vi "Parse.vi"(8 "Error In":errorcluster, 11 "object in":refnum<class "2024_19.lvclass">) -> (0 "Error Out":errorcluster, 3 "object out":refnum<class "2024_19.lvclass">)   [LabVIEW 2023, in "2024_19.lvclass"]
uses:
  2024_19.lvclass
  2024_19.lvclass/2024_19.ctl
  <vilib>/Utility/error.llb/Trim Whitespace One-Sided.vi
  <userlib>/_OpenG.lib/string/string.llb/openg_string.lvlib
panel:
  out "array":string[](array[string])
  out "Pattern":string[](array[string])
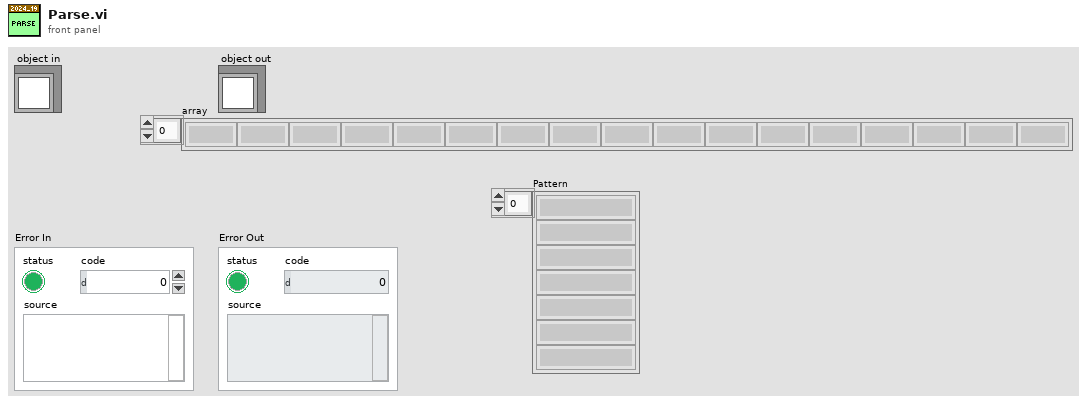
[diagram p1: front panel]
diagram:
  (unwired) "r, wr, b, g, bwu, rb, gb, br\n\nbrwrr\nbggr\ngbbr\nrrbgbr\nubwu\nbwurrg\nbrgr\nbbrgwb" ("PuzzleInput")
  n1 = call <vilib>:"Trim Whitespace.vi"("string"="bwwww, gwwug, ruw, wrbuwrbw, ugugb, rwwgw, wwb, ubgg, rubbwu, wgbuurbb, wrrbru, gwg, uuwwg, ugrrgr, uugrb, grwb, gwrb, buwrwuw, wrb, ruuggwr, rub, guwwr, gwrur, uug, ugguwru, uwr, rwuug, bwgw, ruu, wrbb, wub, wuwgugg, grgwrww, bgubw, wruuuu, bwg, wu, wbrbgr, bgwg, bgrubu, ggru, bgguww, rubgugrw, grwguu, wbg, ugub, urbwuurr, grb, ug, gbu, gbgwurbw, rrrburr, uggru, rubuwrrw, guwgrb, rbr, uruw, gggur, ugwg, bbwrr, ggbbbru, grbug, uuubww, rruug, ubbgwgr, brb, rbbuwbu, ggbrru, uuwugb, ubbgr, bubg, grbb, rgb, rwur, ubuuu, gwuwb, bubgrgr, wuuu, bwwg, urugg, wubuwubw, wgrb, gwggrgu, rwbu, bbbubgrg, rw, ggug, gwbgwbrb, bgugww, ggurrwg, rbbwuwu, wgw, bwb, bbw, urru, ugg, uwguu, wggw, wgr, urrr, urguwr, bbb, bgwbgub, guw, gu, gurwr, rgw, wbb, wggu, brbbg, wbw, rur, gub, rrbbr, uugruww, rbbrb, bwgrgr, rwrurww, grurg, brur, wbr, rgu, gguwr, bwurb, grguw, wuu, rwu, ubu, wbbwwub, urg, rww, bgg, wrwg, ugr, uru, urwggw, buwur, bbrgbwgr, bggbbgw, bbgu, rurrr, ugww, uurbur, brbw, wgwrbr, wbuuw, gwgu, rbw, gbwugwb, gbw, bwwgwr, wurrgwu, wwbg, rburuu, wrruwg, gg, bbbwugg, g, bg, wwguuu, gruwgu, ggrr, ur, bwwru, rwgub, rgwuu, wur, wuwrugw, uw, bubggbr, ubug, gwbbrw, rubgwg, rwbuub, rgrbugb, rbgb, wwgb, brbgw, uwwr, rbrg, uwrrur, uuwb, wug, bwwgrgb, rg, wuwww, bgrb, uurgw, rrburg, wubg, rwrwur, rwb, wrw, bwrw, wg, wwgrubwg, bugb, uuubguuw, gruu, wggruuu, urwu, wuugb, rrwww, bwrugbrb, wrgg, bru, ggww, wrbrrg, ugbu, rwwrrguu, wrg, buguu, ugbbww, urwur, grr, uuw, rrub, rb, bww, wgwr, ubb, bbbuub, ggbrw, rbwb, ubw, uuwg, wgrrbr, grw, gwu, wuwwgr, rwuw, gbbr, bguur, gwgrrw, bbu, ggg, grg, urbwwrr, bwgbuw, bw, gbrw, wbwrb, rurg, uurg, guugb, uww, brrbggbu, ruww, ru, rwguw, wgwbug, wwu, wgwwbur, bu, rguu, uwwwg, rug, wwg, brg, uwu, ubr, burg, ruug, rwr, uurugu, gr, uwubu, rr, rbwrbw, gw, uwwuu, ruuwb, rbg, wwrw, wruubg, bgwgrwbr, wuru, ggrgr, br, rwuu, grgbgg, urw, uub, rgrbb, wbuwb, wgwbg, ubwu, gwb, uu, rrrr, rru, gwr, uuubu, grgw, gbb, gwug, wbggwu, gggr, wr, wuw, wgg, buw, gbuwrwu, gb, uwb, bgubgb, rggbbbu, rgubgggr, rbgr, ruwr, wwr, grgbrb, ugrubr, ubgu, ugw, ugrr, ubg, ubgb, urb, wgb, wbwrbw, rugrr, ub, gbr, bugrg, ugu, rgrw, rrrrurr, bgbw, wgwg, guu, wrrubu, www, wrbu, bgrguwr, wwur, ubgbgug, wbwu, buu, gbgubrw, b, ggr, rrg, wwwb, wgrrrw, ubgrug, rrr, ugbb, wugubbur, bgwb, buwww, ugb, buub, wbrru, wuwguur, gwrggg, bgb, gru, bwwr, bgr, gbbw, wuruw, gbrgu, uwg, ubrg, ggu, bbwg, ugrbug, bbr, r, ugbwub, ggb, bbg, bggwb, bub, gbg, burbr, brw, wbuu, gugbb, uwubg, gbgwr, bgwwru, rgugb, uubgr, bb, gug, rggb, wugub, wrgu, wrwguug, gur, wru, bgbr, bug, bwu, ubbur, uurugb, ubgug, bgrr, bgbb, uwbrrug, bburur, rgr, brbbrw, rrrrwu, rgg, urwuwr, wwgr, bur, rugwg, bgu, urbg, wwrgbuw, rrgwrbb, uuu, grwgg, bwr, wrbrb, wrr, uwuuur, rrubu, ugwrg, rwuwg, wgu, rwru, rrww, urr, rwg, bgw, rbb, bgbubrg, bwbb, u, wggurggu, bubgw, ggw, gugg, ugrru, wbu, rggrrb, ubrgggwg, bwuu, rurb, wgrrg, brr, rubr\n\nwbugbugbgrgwubgrrgrubgbwubugrbrrubgwggggubrrrwrbr\nwbgrbrgbwrrurrrguwbubburbrwgwrbuwrbwgwuwubwurggbrggbr\nurbrbuwgbgwwwbgbwrugruburguwgwbgrugwrrbwbubgrwgww\nrrbgwgrwbrbuubbuugrurgbrbrwrbrggurwgwrbuwuwgubuwwrru\nuburbwruugurrbwbgbggrgrrurrugwuwggggubuwugbgurgugurbbbu\nwbubwwubrurggrrbbbuuwuwgggbguubwuubbwggrgubwbuggrbrrubg\nbbwbgggrwrrbwurubbrgugrguwrwwrrguurwwburgruwrrbrrbwgbggw\ngugrgwgbbwguuwbbrgwrruuuruwgbrurwubggbubbgrugubgbuwwgww\nbbrbbwgwwwbrgbrrgwgugwbwwrrbbwwgrwrrrrwwgrbguububgwrgww\nubuuuwrrwgwwgbguuurrgwrbbuggruurbwuwrubuugrwuuuwbwgubbuwgww\nuwuuwwwrrruggbbggrgwbbggwgurruwwgrugwrgww\nubbbrbbgubugugggugrbwuwbgbbruguburwugrubug\nrwwruggrwguwguwgguruubrggbgbbubwwrbbgbwbwwbbubbruwb\nbrubrbrurrbugwgrgrruuurrbgguwuwubbggbwgurbbuwugur\nwwrguwbwuggubgbrgbguburugbbwugrwwwggwwgbrgwrugrwuubgwwrggw\nuuugwubwgwrbuurbrwuuuubwgbubwbwrgbgrrbbggrwbwbg\nbrgbbrugbwbbwbuugubwrbuggruubrgwwuggugbubbgub\nurbrwguurgbbrgbwrugggwwgwubbguwrurbwburrwgu\nuwrbgggguruwubgrruwrguuuubwugwwrgbgubwrwguubuubwugwbw\nguugwbgwbrgurbrbwwrrubbbuurruuubburgrruwguwwwww\nwuugwbwbrgbgubgwuwwbggbubrugubrgggwgrrbrrrbuwgbb\nwgwgwurrrbwbwuuwgbwrggwruuuwbuuuuwrrbrrbbugwuubrwu\nwrbbgbbgugbbwwurruuruguuwuwbubbgruwurwruggruwbrbbwbwwbu\ngwbgwbbwwwuubrubguggguwbguuwrubwbrgwwugwbuuwurwrgurub\nugubrbubwbruubwugugrrbwbuggbgbrrgbrrgbbbgrguwwbrgww\nugbbburwwwbrrbrwbrwwbrwwubrrrwwubwgrrrbbgrwbbub\nuuuwgbgbuwguururugrbbbwuwurbuubuggbururrgbwuwwrwuuguuugwgww\nrwrbrgbuggwwbggwggrrwbgggwggurrbwbbubrgbuggbbrrugrbwwuwrrgww\nbrggrbgbruwrggwbbbuwubuwgwbrwgrwrwrwruuwggwrruwgrbru\nbuwugrgrbggwrbuggbubwwugugggbbrggwugbugburgrrbgbuwr\nurrwwwgwrbgwgbuwrggggrgbburwgwuuguwbwrrbbwwbgbwrwwwwwgrgww\nuwwbgwbbbggwbbbrgubrrrgbwwrwwbwbuwurubgww\nbbrrurwwggrbgwggrrggrrgugbubwuwbbwrbrgubgggbgu\nwbuugbubuwbrugrwgwbrrgggrubrbrwbgrgwgbrwubgrgww\nggugbrggrrbrgbbwguuruwurggbbggrbugbgwrbwbugbwwuurwgbbggwub\nurbwbubwurrgrruubwurbwwrwuwguurrrgbwgbwguwrgbgwwrwrugbbw\nbbrgwuubwrgubbrrgrwgugbrbuwuwuuurwgwgbgrbubbbruuubgwg\nwwbwbbbwurgubggugrbwrrbwuugugwbrrwuwbrwbrrrbrwbbbgrrrwgwgww\nuwwubwgubbwwugrugbwrugwbrwrrwbbgbugruwbwggruguubbrw\nuuruwbgwbwbrggrbgrugbgwwbbbgugurgrgggurbwrrwurguu\nbrbgrruwguugwbuwubwwbgwgbugbgrubrbbubbwubbuggbrgbrwugbrwwgww\nbrwrbwugubuguuuggrurbwruugguwugwgugwrbrbgwwrbwuurwwuur\nbbbguugubrugurrrgugggwbrrrgrggbugwwurrgrwuguwgbwrbgwgwg\nburrrgruugbbugrwgbrwrrgrugwrwrgbrrbgwwbbuubgw\ngurrgwuubbruwuwgbugbbbrwuwgbwurrurrugurruugrgbbrb\nbuwurgurguguuuurbrrwgwgbgbwubrgrrrgbrbuwggwrurbggurb\nwbgwgbgrgbwubwgubbbbrggrwwgwuuubbbrbwburgww\nbgrugwbgbwwwrugrgbbwwrrgurrbwurwurggwbwbbwbruu\nwbrwggwrwbggwwurwbububbuwbwwuwwurgggwugbbuwgurruwg\nububrrrruwrwburrggbgwwbururuwuurugrbrrrwrbgbb\ngbgrwggrguwurugrrrbbbubwrugrwubuwurwuguggwwrbr\nwgbguuwbbrrrgruwgugrgrwgrrugbrgrubugubggbrbwwrwwwwguwugu\nrwuurububuubburbwwbbuubbrgrrbubbwgbwrrguwrrbubrgggwgww\nrrrburbguwrrgrrbgrggggrbwgrbgrwbbbggugbubrw\nggrwgwubbuwrwruwwgwwbbwbgbwggubwgbrrubgww\nugwbbwgubbwurwbbrrbubugbgwwbubbbrgbwgrugrbrrbwgww\ngrwwwggbwuwrguugrbgrggbubwbbgguwuguurbwgubwuguuwrggwwr\nbrrwgbuurugrbuwguwuurguwbbwgbwbrwuubruwubwgbgbg\nubrgbwruwguurrburgururuburwwrrguurubuugrbbrbggrwbuuuwrrgww\nrbwgguggbrbgbgwgrgrggbgbuwbgububrruwrbrgww\nggrgwuruurgbwururwbbbrbbubgubugwubbbwrurgburg\nguuwbwgwurbrugggrwwwbrwrbbggwgugwubbubgggu\nwwggrbwgbgbrwwuwbwurgwbubbggbbgwrrggggrbwgugb\nburgburgggbgrwbrrrbgwgbwwbubgwwbugubgwgbwwrrwwwrrug\nugbbbrwbgruuwbwwggbwbguubrrrbgbbwbbbgburbgww\nuuburguubgubgggwbwggurgguwbbrgbubwuguururrbwrg\ngubwuwubrwgugrwwwuwbrgurrwwbrggrbwbggwubgrgruw\nguwgrbruruwrbwruuwggrwwwrburgrbggbwugbgww\nurwubuwuruubggwwggwuwwggrbrgburwrbruwrbwrrgww\nuuruugbuururbguururbgbugguuuuwwgguubwruguwwgww\nwgrbguguwgwbguwwbwrrwrwgbubrgurrgwwgwruuggwbwubb\nwburburwbgwrwgwwwrwggrwwurrbrrruugurgubrgg\ngbguguwwburwgburrgrbgugwgrwrwruwubugbbgugbwggrrrgww\nuwgwbruwuurgwgrgbuugbgurwruwrbbugggbbuuwrbg\nubgbwbrrrbwuruurggugwubruwwgurwgbbggwbbwrrwburbb\nrgwuuggrurgwwuuuwrruwggrgbwwbuwwbbwurrbggwrwwurrwgww\nrbgubuwrwuwrrbbuugwwurruugbuwguwugwrgrgbwburrwub\nrurbrrwugbwgwrrbwbwrrubgwrugbwwuggbubwugwrwbuuggbgrrb\ngrbwwgbrwrurwbwrbgrwrwuwuwburbrwbwugwgwrwgggrbuwb\nugurrgguwbbgbgbgggbrgwbrwwwrbubuurbbwwbgrgww\ngubuugurbrrburwgruuuwbbruwuubuggwwwbrwwwbwwrrggwb\nugurrbrgwurgrrwubbgbwwwbgurrruruwrbwgbrbrruuwuwgwwwbgrggbgww\nbwurwubwuruwggguwugrrrbwrubbgbuguguwggbwubrwurbwbrwbugwbu\nrwubrbbbuuuwuurrbgbugggwbbgbgwurbuuwbruurguggbuuwrrrubwuug\nwrgwrrwguggbrwrbuguruwwrbbbwbbwgbwubururubwrwubrw\nbuwguruwgrwrwwrbgbbrrbggbugwrrugrburubgbggrbbwubwbgguuwubgww\nwwubrbrgwrburbruurgurrgrbrwbrbuwugurbwuubwgwrgbuwu\nrbwrggwgbrbrrgbrwuwrrrrwurbggwwuwubuugwbugrguubrw\nuruggbgubbrrgbrbwwguurggbbugugrrggubuugwwu\nggbrwgbbggbwgwggbbguurgbgbbbubugbbgrugrgubbu\nggbggwbbrgurwrrrgugbgwbgwwwugguguuugrbuwbwbwbrbbgbrbgwur\nrbwrbugwrwwwrwwugbbrbrubrrgrugrwrwgbuubuwgwuwgrrrbgww\nwgwwrwgwruwgbbbbwgbbgbwgwrwruwwrwwuuurgrwgww\nwwgbbuwguuuwbrubbbwrrgbwwrguuggwuubuuwubbruw\ngbgbbuwbrwwbrurgwbugbwuwurbugbugwrwgwwbwwuwuwbuuuwr\ngbwubuuwurbuwbwuuguguwbwgbgrbgrgburubwbruuub\nrwwrgbrrbrbbbrgrwgrgbgwwgrwbbrrguwbwwrgrruugrrgww\nwrbgbrgrwuwwgwrbrgwbubwuwwguuuwurgbbrwgwrruwgg\nuwrbgrgruwubggrgrguugrgubbwrbwwbubwgugurrbgwrugbgw\nbugguuguwbrurrbrggbwwguubrggguuuwgggrbbgrgbrubbrrgrugwwrg\nbgwrwbuuwuuwrruwgrrwbuwuuruurgrbgurruwruwr\nurrrrbwrrgbuubrbbgggggubuwbbguuwurwgbrbgww\nrrbgwubrwbwbuuuguuguubruwrurggwgwgrrgbwbrwurbwbwgrwrgurwwg\nwrwurgwrgwgwwuurgrgggguwbgrwuwbwbwrgbbbbguugbbrbrruguwgww\nubwwbugbwwwrrgrbuwbbwuwubbggruuwrbugruwbrbbbubrw\nrrbrgggubrbwrrwrwbuubugrwbgwrurbugubwbrubwrbrrbwwbr\nubwbgbgubwgrbgubrbrgurrgrwbgrgrgwrugbwuuwgwuguwwugwgwururg\ngwwugugbgwbgggwggwwuubwwurwbbbrggbuuwgbrrggwbwwbbbgru\nbgwgbbuuwbrrgrbbuwwwwrwugggrgwrgbubrgbwgrgwgruwuuubgrw\ngruurgugwubuwbbbrbgrgwbgrgggrrbuwrbuwbruwwwurbbr\nrgrwuwbwbruwwrrwbgwwrubuwrrwrrbbrrugrubbrgbwwurbrwwgww\nbggwwrrurwugurgrwwwbrrggrrwgwgwgrbuuubuguw\nbbgbuugrgwruwgwubbrbuurbruwwwgwbrugrgurwbgwugwwbrb\nurbbggbrurrrrbrbbuuugwgggbggwugggbwwbrgbbrubw\nbgguuwrgrwurgbwwubwrggbbggrbrrurwbgwrgguubgurrggrgwbggbg\nrgbuwrurggubbugwbubrrgwbbbrubuugubbguwurwguuuugbu\nurwuwbbgrgbwggbrbbbbbrggbwwwgrurguwrgubrgwrbwbgwwwgww\nbubugwgbwwuwwurrrbububwuwbgbbggwubrbbuwugrwuburgrwgbugwr\nbrwbubwurgwbggguuwurrbugurrugwrbbbwggbgww\nruguwbrrrbgbwwuuwwbgrwwugrrbuubgrwburwuggubr\nrrbugrbrrgwruugrgbrbuggbruguwbwrubbruubrrrgbgrgwgbgbb\nbugggurrrrrgbuwbggbwgrgrrbwrgrgrgubuwwurbbwrggrwruwg\nrwrggruurbwguuguwbbrwwgrruguuwrrugbbggwgbbuububur\nbrbggbwwgwbbruubuguguwbruurugwrrgbgbwwgubguwrwuru\nwgwurwruruburruwwwgbgbbwuuwbwgurrgwurwbbwrrwwu\nggubruuuubggrgugubugrgguwwgguwwwuruuggubbuwrru\nbbbggwrbbgrwuwwbggwrbwbrwrguwgggbwbbrgbuwrrb\nwrbbgwgugrggbrwwwbguurwrgbrrwbguuugwrbwubbgwwubrr\nbbgbuwurgbgrrwbuurwbgburgwwbbubwggubrburbrbgwrrbwrbuwgug\nruuwrguruburruwwrugbwwrubgrgrruwruurwwwgrgrurr\nrbwwwwubwrwrurbrrwuwwbgruuurbwbrwgbrbubgwuubwurgww\nugrbgubuuwwwrbggrrwbbuubwgwbgwrubwgubwubuwubgwuubwruwu\nwwwwbbrgbwgrugrgwrgurwwuruubrubgwugwwggrrgg\nwbwbwbrwuugburwrgbrbrbwgbwbgwwuruurwbrbgwuuwbr\nuubuurwgbrubbbwbgrrrrwuuwgwggwgwwuggggbuurgguuwgw\nbbbrbgburggubrgruggggubbbubugbbrgrguurwbugb\nurrrwbgrburwuwuguwbrubwgbrgrwgrbrbuwggurgguwrgrugurbwgww\nwuggrrwguwwuruugrrbwwgugurburgugurwgrbwbuuwwrubgwgbwuwu\nbrrrgbrrrwbrwrbgggbbgwgugwruwrwgbbrwwbwrrbgbburgww\nwbuuwgbguurgbwuuruwbgbwuuuuwbuggbwwurbwubgwb\nuggrrrgwbrgruwrwgugbggwgrwrbubburugbwuuwrwbgugwwbwrguwrwrgww\ngbwrrbuguwwwubuuguruurbbwbwbbuugwurwwgbuurbbwugrubrbubbgww\nbgrrwruwrwbbwgwuwruwwgbbrwgburbrrrrwwwuwrbgrrbrwuubgww\nubgrgwrgurbgwgwwugbbbrrwgwruuurrwbubwwugurgwggg\ngrubgrbgwrbbbbbubuwwrwrurrbbrrbububwwwwuuub\nrbwrburbgbrbrgwwuwwbgubrrguurwugbugbuggubrwwururrburgurgb\nwrwgurbrwgwgwrwugrgugrwbgbguugbbuwrwrrbwggbbgrgwuu\nguggwgbgwurbbrrwrwwggrwwgrbubgurgwwwgrgbwwbrwwuwwwrruurr\ngrwubwrrubwwgwbrgbrwwwgbbbgwurrbbrrgurwwuwwubwbgubuubugrrgww\nurgggugwgwurwwbgbbrwbuggwrggbbbbbwuggbrbrruu\nrbuuwwwurugubgbgubggbwbwrrrbbbggbgwggggguwwrrrwwr\ngbwrubwgwrbwwbguwuwbwbgurgbruwrwbrwwrbrggurwuwb\nuggggwrurguggrbgbgrrurubwggrbgrggwrubbwwbbrbwrgwgbuwrbw\nubrwurwuuguuggugrggwwwurgwrgbbubrugbwrrwuguuwruguwbgbr\nuruwbwuwbggwgwrwugubrwgbbbbuuggrbbrrwrgww\nwbrrrugbruuwgrrwbbwwbrwugwgbbrwrubwuggbwburgwuwwbrubwubwrgww\ngbubgrrrbwbgrbgrubrrwugwugubwurwbbrgwrugwgrbrgbrrb\nubrgbuwwwgrgwbuggrrbuwwwgbwbwwrwgugrrrgrwguruggbbbrrugwuuu\nrgrbbwbuwrrubgbbgurbbuuuggrgwrrrrbwgwbwurggwruwgbrbggru\ngrrbuwwuwwruurruuurwguurubwbrrbuwrwguwuwwrwbwbbgbwugbgww\nwrubgbugbgbubgguggugbuburwgbggggrwgguuuwwb\nrubwbbgrrwwbbgurbguugrwgrwgwrbugbguwbgrgrgrwwgurg\nugrgrurgggbgbgbruwuruwbuubrbggggbbbugrurwgrubwur\ngrbubbubgwgrggrbggwrbuwbwbuurbrgrwrbubwguwubbwuggr\nbuwgurrugbbgwwgggbgwrbrwbugrgwgwbwgwuwgrbuwgwurrwwbguruwr\nwrrugbgwuwwwubwwgrugbbgwggrgbbwgwwbuuruuuuubguwrgww\nurubbbrrwgugrgurgwuurubrbbgbwbrrrrbbwbrrbwrwuugbbbrgww\ngwrwbugrbggubrrbgwggugggrwgubuuwrwwbrgrbgrgurbbwurrggrurb\nwgbrwwuwwwruuubgrguugrwuwurbrggurbrbgwwbbg\nwgbuwubuwwuwwwrbburuwggwgbbwwuuwwrwubrrwubwbbbuu\nwurbggguurgwwwrubbrwgubruguugubrrbggwwurbu\nubrrwwuuruwwgbruruuuuwgbgrrgwubbggugbgbwwbu\nwubbbwwbubwggburuugruwwuwbrggrubgwrrbuwgww\nwrwggrruwugrguuwggbuwwgrwuubbwbwubrgubgggrbwb\nrgbbwrbbrwrwgrrrwubwugrgrwwbrwrwuuwubwbgrgrbbbw\nbgwbuugbwuwbuuwugrurwrbbgrwbbgurwuuurbuwbwrr\nbuurguuwgrrwgugwgbwgwgbrwwwurrgrbrrwgbbbgruruurbbw\ngurwubgrguurrrggugruurggurggwurwbgrwggwwbgww\nrwwbgbggrrgwwwbuwgrbuubrgbbugbuwugrbuwbbwgbbrbuwg\nggrgrbruwrgwwgbgrggwwbuwwuugbwgugguwrrbbbgbgrbuguu\nurugrwbuwgbrrrwgrbbwwwubwrrubbbrgwrbwuuwugbur\nbbuggbbuwguububruwurwurbgrbuubugbbugwbwrrwrrubw\nubgrbggrbubuwwbguguurgbwguwwbugwgwwbrwbggwguugwbr\nubbbubgrgggbwwwgbbuwbwwwurgrgbrrrbbbubrrbbrwwgbbbgwu\nuurrwuubwbbuwrrugbgbwwbgwugubwuugwggwgggwrguggruwggrgbwwwr\nbrwbwubruurbugubuwbwrggbgbugrgwuubbwbgwbuwggubrwwgub\nugbugrururugrgwubbgwbrwwrwbwggubuuburwurugrgr\nuwubgwrgwrugububrgrugbgrgugwwggwbgrurbuuuugubww\nbugwwubuwubwgbbrrwrwwuwugwbbbgwrwwgburbbrubw\nwburggbbuguwuuwwuuuwbgrggbuggurwbuwuurrwwww\nguwwubrbrwrwuubuwuuwrrwuwbgbubbgbgbggbbbgurbwrrurgww\ngwwwrgrwwbgrwrbuurgggrubuguguwwbbgrwggwrbgbggbubrwwwwwr\nwbubrgwrrgbbbbwurwububuurgbrwggwuwbgugurwwbb\nrgrurgugurrrgrrrbgurguuguwburrubgrrbwugbrrubuwbgww\nrruwwuugbgwwrruwuwrubwuggwrwrrrwwgwgwuwbbrrr\nguwubbguggubuwgwuwbggubrwgwgbwwgwrwgubbwrrggbuggruuruwgww\nuggbubwbbrrbrrwrgbwrwbgwguurrrggwwgrggrbgurugb\nuwurbwwbrbrwbbuuuuwrgwgwrbgguwbrgwburbugwrrgggbrw\nwwbuwwrrrwrgrgbgurggguubburrruuggbrgwbgwbbuuguwbr\ngwbwwuwbbrgrbgrwwbugwwbubwwbwuwuwurwuurwubrggggu\nwrrwwguugugwwwwgburgwwgbgrruubuwuuwwgrwbur\nwrbwbrrwrbbwwrgrugbwbrugrguwuuuwgubwgrgggwwbg\ngbbrgrgwurubwwwburbggwwggrgrbgubgwwbuwruwwb\nuwgrguuwggggwgwuubbuwrbbwwbwrguubgbuuubwwwwrugrurgbwg\nwuugbbbuguuuubguuwwgrrrrwgggbuwrwuruggrwrgu\nrgwrbwgwrrgguwgwrguugbgwgrrubrwurwbrgbuggwuwr\nrgbuwrrrbwuwggrbuwwruwwurrwuubwguubgrgrrrurrgrruggrr\ngbwugrurrbbubuurrurgrggbrbwubruguburguurrwgww\nubgwwwwgwgwguuwbgggrbggwbrgbuwruwwgggwgubrrgwguuwugggwggrgww\nbrrbrrbrgurwbgubgbruuurgrwbrgbbbrgruwbuwbrrg\ngugwuuwbrwwuubugburbuggbrwgrrrwgrrbgrurrug\nrggbbwbbubbwgwrbrbwwbrbuuuurwubuguwwgrrwgrrwrurbrwwbrbw\nwugrrggurbburuwwrgrgwrgrbbwwuwgubgggggrgww\nurbrubuwgwubrwwbggguguwrgrurgbrrgbbuuuuruggrurwgrbubggwgww\nwgggwwrbbrrgugwwwburruwrrbuwrwruugggrurrbrrbgururg\ngrgwggwgubuubwbwbburrwwgbburbgburubwwrbwbrgrw\nrbrbubggbbwwwwwbgbbuurbbrgugrgurgbwgwgugurruubbburggbgr\nuwuwwbubwbgwrwwubwuugrbwugwgurgbwgbubrrwbbbwbwbbrwgrrrubb\nbubuwgggbwurbwrrwguubrbbguggbrugwwbbgrgwgurbuggbbbwu\nguguuubwgubbrwbuuugbubggbbbwrrgrrwuuwwbbbwbubbwur\nruwgugwbrbrwuwwgwuwubuwubwwuuwrggrgrruubwwgww\nuwgrbwuguwwrgugwgbgbgrwbrrwguubwugbwbubbugbwg\nwrwruruwbuwrrbbuuuuggbbgugwrwgbguubguwrwuwbruugwbrggrrbgww\nuubwwgwrbgwbwuwgbuwuuwguwrwurwwgwgruuubgrurubguwurbbuwb\nbruuburbubrbrgggrrgwuuuburbrrruugbrurwurubgww\nubrwwrrbbgrburbuubgwbbwbgwrubgbwbugbbbrugrrrgbbubugbubgww\nugggwwgbwgbbbwgrrbruwgrrgbgrgrggwubwuwugwgwubggb\nggwrwuububwgugbgrwrwwurwrgwbbbbwwwwubgww\nwwggbwgwbuwwwbbwwwwubrurbrgugrgggbbwgwubugbrrrgguguuwb\nbwurwugbwgbubgbuugrwbrgbwwuwgburubgwrbguwrrwuubuugwwwwbg\nguwbgbwgurgugrrubgrbbbrgwwwbruwgbrwbwuguuubb\nwuubbrgggrggbuugrguuwrgrubgggwugruubguuwbgbuwwruruwguggwrw\nurbrrwuuuuburwwwgrgurbwwwwbbwwwuwubugwuwggrb\ngrgrgwwuuwwrwwrwurubburuuwrgwruuwuuwwwrwrrgbgrbwurugrrgrgww\nuuwurggbggbuurbburgwwubgwbbgwrbwwuwwgurggguuubwg\nuubbbrggwggwrbrbbrwrgwgrbbugwuurbbgrwruwrwguwrwubwbbrrgww\nwbwbugbrbbwuburgurwgrbbguwurwwwguwurwbrurbggwgbbrgr\nubwgbgbgrbwburwgrwurwbgbgrgbrwrguwruwgguwwgwbwbgrubg\nwruububwggruggbggbwggrrwuuubguuwwwgwwurubrgrwbrgww\nbrbgruwgwuuuwwgrwguurruwurbubgwgbwbuwugrgrbuuuwwgbwbwgwwr\ngggugwbwbggbuurggbwbgbbwrugbrbwrgurbrrubrgwu\ngrgggbrruwgwurwgwrruwgrrwuurrggrrwugugbwugwurrbu\nbrubugubruwbwrwguwrurggrbgguurrwrbwwrwrwbrbrugwgurbgguwuww\nwgwubuwgwubwubgugwbwurbgwbuwugbbubuguuugugugrubwuggrrgrbgu\nwwgbrbggugugwwgrbgbwwrwrrruwuugrbugrrrbggwgwuwwwg\ngrwbbguugugrgggwrwuwbwwugurbwbgrbwbgubgwgwugrguw\nurgrurbbubgrwruwrguugrrwrbrggwwbruwbbwbuuggwrwgugwgww\nuwuubrbuugwwbgrgbbgubrbrrgbbguugubrrrgwrbbrg\nurgggbuwbbbwgbrguuwrgbwbwbgrwburuwuwguurbgbbur\nbrbbuuggbwugrgbruuwgrurrbrbugwubwrrwgubgbubgrwbgwrurwurg\nbwwgrubwgwgrwuruguubwbwrguwwwggbrubbwubrruggg\nuwgrgrrrggurggrrrrgbgbbbgubbbrgrubuwrrwgrrrrrwgrbwwuruggb\ngbruuwwubrurugbwrruwbrbbgwgrrgubrrbrurrwbr\nwrwbubuwbruwgrwgbugwrburrrrrrwwrgrurugrurwrrbrbgwb\nwbgrwgwrgrgwwwrbrrugbwwgggruruwrgwbwrwbubwgbrrbgru\nwrbbubgrgwrwwggrwgrbbuuwbwbuggrwurbbrgwwbbbrbgrbguub\ngbrurwrrbbgbgugbuwrgubggrurwrwrrrgwgwwwuuuwruuwgww\nbbwuwgbrgurwuwbbwrwuwrwbbubrgurwbrrwuwbbwrgwbwbggrgrwu\nwggggwbgggwgbwurrgbbwbwrgwuurgurrububgbbbbrgrwruw\nrgrugbubugwrwrburrwgrrrrrgwububwrruuuugbgwbwwbbgrr\nwgrruwwugwuruwwbrwruruuwgwbbgrgurgubgrgugwuwbwuburrwrbubwu\nwuwbbubrgugbgbuggwgurubggrrwrwrwgugurrwrbgubugw\nrbbrruuurgwrugwubbrrrbwwrwrbgwgwubuurwgrbgrgrbbruwrgwgb\nwwuwrugugbwrgbwgbgbuwrggruuubgurrubuwrurwwgww\nbrurbgggwrgwurrgwrbggrrbbbwbgbrgbwbuwugwbbgwbwgww\nwbgbggguwwbuggubuuwurugubrbwrbwurugbrrubrrbwbbbwgu\nwbgwuurwgubrrgrgbuuuwrrrggrggurwurwrrwrggrrbbr\nwuwgguuggrgwuwwbgrbwwrbuwrbwbguuwubwggbubgww\nguwrwrurgwrgguurrrbugwgurwrbwwubgggbugwgww\ngrrrbgbugwwggwugbbrrwurwgrrurbuubrbbbwgburgurbwgwwrbgwubgww\nugrrugwbrwbguwbbgrgbugwurgrwbrrbububgrbwgguuwgbuurbb\nwgugrruugbgbwbrrwgbgwurbwwgwwwggrguubuwgburugugbbbubuuubrw\ngrbbbubgrgwuuwruwwuwgugrwugrwbwguuggwguugggwuwubrwbbgubgww\nwbubuggwbwguwubbrubrgrwgwugurbuwguuuwbruuuuurbburugw\nrugwgrbbgurbuuubgwwwgrgbgggggbwrbwgrwurrrugrwugrubrgbrgww\nburbwuguguubrugwrrwurrwbggruuwwuwubgbrgww\nurubuugrrbrwwbbrrrbbgrgbgwgrubrgwurbuugwuburrgbubb\nbbrgrgugrbgbrrububurwrguwbgrbbbrbgbuuugugbwrubrrg\nbbrwrburuwgrugrrwuwbuugwwbgurrwbrgruurbbgwb\nwbgwwgubgrrbwbwbbwuwubgbggggububwuuwwururrgrw\nrguurbrguwrrbbwurwgubuwgwguwrggwwuubbwrgwrrurwugguw\ngbgbrubuugwuuwbwubrgggwgbwwgwbrrguurwuwuubwwuuwuuuwwrwgbuw\nuburuurwbrrgurbbwrwuwwwgwgubgbuwuurguwbgwggurbbbbwgww\nwurrugwbbrruwrbbrbgguuwubburgburrrrbugbbrrrwbrbrgwuu\nrbwbbuwbwrbrwubgrgugbrbrbgubbgbgwwbuuwbbrgrwggbwu\nwruuurburwgwwubrwuwrgurrbbrwwwwwbrwwwbbbrggbbubbugbuwbgww\nggugwwwbubbwurgurbugrubggggrrugubrwwggrgrbbgbububbwwwg\nrwbbugbggbgrwgbbwrwwbgrwwwrugbuwuubuuuuwurrruwwwwggwrwuuu\nwubbuurgrgbwgruubgbugugrwurbrgburubgugrwwrgbubbgww\nwuuruuwubwguuugrwwrbrrgbrbwbrwgwubuwrrwubuguurwwrwgww\nrgugbwrgubbgrbrbuwwubgrbbrububruwrbbuggbruububrubgugrw\ngwuuuwurgbrgwrgguwwgugbbgurrbbbgwrgrggwguwu\nwwuubrwwrwrbrugbwrbwuruwbrwrugwbbuuwrrrubuugrrwrwwgww\nbgwgurwgwbbbgrwbbwwgbbgwuwuuuwwrgbubwgubbrgrbrwbgrgww\nubggbwrbwbwwbrbbbrwgbgrbrwbbbgwgrrwrrwgww\nrwubrubgrrrbgwggwwbrugrubuuwbrrbggbuuurgwggwrbwgwuwugrbrb\nbuurgguruuwuubggwrrruuwbbuggrbururrbubrbrbgubrwbbgrrgbu\nguugubwwbwgugwbrggbbgurgrwwrguwrrurgububbbrbguu\nrburuwbbugbubbgurrbguwbgrgwbgwbrbwwgbrrugbugruggrgbu\nbgwubburubruubguugbrgwgbbrrgrrurgrwubuubbrurrrw\nrugurggbgbgbbbbrwubwgbguwrwgwgwgubwgrggubrrbb\nwwwrwbrwuguuubrbbubuguwuugggrrgwggbbrrwbbgww\nuugwuwugwuuugrwuwbwrubugbbrwgrrwwugbrwrrurrurwgrwurururgw\nrggbgrgrburwurggwwbwwwwugbgbgwwrwgubwbwuwwrgbrw\nrrgburrgubrbgubbgbgrurburbwuurrgwuururwgbuwrurruwbururu\nbburburrurwbrwwbwggggrgwugrwrbgggburubgrwbgwwwwwuwrrrbb\ngwrgrrwwuwbbrubbbwububwbbwwbguuurgwbururwgbgww\nurgwrwrgbwuwguuurugwrbgbrgurbuwwwbwgwgrwrbwrguu\ngubgbbbrbwbwwrbbgbrrwrbuggugwbuwbuubbubrwwwbbwbgg\nrgrwrgrurbuugrrwrrgrrgbbwgwubrgbgbbgugbrubwbw\nbrbbwwgrrbuwubwrbrwbuwwrrgrrwbbwururgguwuubwrggbruuubbb\nurrwrgbrugrbbbwrrggwugbgggbgbrbrggrugwbrruubruwbbb\nbbbgwuruggbwrbrbwbrrbgwgwwbbgurguurbrgrrugwuguugwurbuurrg\nbrwgggguwwrgrgugwgrbwguwrggwuuwbguuubrburuu\ngbgrrurbrrubwwrwggrrbbbugggbrwbwbwwubbubruuwgur\nrwbrwgbwrurgurwwbburrbuburrbuubrwgwwggww\nrgbwwbrbrubrurrguwguuwrbbgruugggbgugggubgbwuwu\nuwubbbwuwbgbuubbwubbrrrubwurwgbgwurrrgrwwwugggbgww\nggrwwuurwgwruuuurgugurrwwrgwgubrrgugrbgww\nwurbwbgwrwrrwubuuguwurgwgrgwguwwuuggwbuggrbwgww\nrgwwgbwurbrrwrwwuugwwbwwwubbbgrugrubwgguwgwbur\nrgbgurubuguwburuuuggbburuuurwugbgrbwwuurwwgurggbrrgurrruw\nuuurgwububbruwwuwwbggugrwrbrwgggwugwbguggrbbgrrrbr\nbggwgwuuurwuwuwgrwwuwrgwwuwrguwggwuwwrwbbugwbrggbrwgww\nrbrbbbrrrgwrggbbruwuwurrwurwwwguburwgguwbgwgww\nurggwgbubuuubugrbrrubwrbgbbbugwrbguugggrwgwubgwbwg\nugwbgbgurbgwbgrwrrbwrrbgbwbgurrrubwgbuwwbgwu\nbgggrgbrwrruwbgbgwbrwggggrrrugbuugubbrwubbwbburbgrur\nggbgwgwuuwurwrrwrwbrwgwrurbrubwbbgrrbgggwgg\nbwggugbwwruwbrbwrrwrbwbuwwbuburwwrrbwwuguuugw\nrwbuuwuwburbgbuwbwwrbwgwgrgurbwuurrbrrgbbwrruwgrgburbgww\ngwuwuurwwrbggguwruguwbbwugrrgurruwbuguwugbrwgrgrgrbbrwrbb\nbrrgwurbuwrugubwgurbwubburbwggrburrbbwgwbgu\nuwgwrrugwwurburbgbrbuubgugrwurrubrwbbbgbbugwbububuwb\nwbgurrrurubggrurgbbwrbbbbwwurwuwwggrwwrbbrbbuuwgwbwr\nrgrbwgrburwwwurgguwubrgbbuwrwubggwwgwgrbwgwugbwww\nwuurgwgrugrurwgurbrgguugubrbwugrwgwbugggbwgbbgwbrrbbbgr\nbrbuwuurwwgwrgwrwwgburrurgwrurwrrbwgrbbwubbgwrugbrubgww\nrrggwwgbwbuubuwuguwugwguwuggwruwugbrgbrgrrgwgww\nwwgguggwgbrbrruwbubwgugwggwwwrggrggbubbugbruw\nggubrwuwubgrgwrbbwbbubbuwgwugggggrrgugbbggbgwurbwrwwgww\nrwwrwwwwrubwuurwugrwubrbubwuubuuggrgrwuubrgubgbuuwgbugwgg\nrwrbburrwrwruubrbbbbwgurwrgggwwuwrbgwgrgrgwwbgww\nrrgrbuwururuwbruburburguruggbugurgrrrgbbbugwgbuugurwwu\nuuuwgrbuwbrwwurgwrrurwurbbbuggrwruubgbbrubgrurwguuubgr\nubrrgwbrgggbwbuguwubgggurwugugugbbrruwbgbwwrururgggbggwub\ngubwugrrgggggbwgrwruwrrgbwwuuwgwgbubrwgrrrgwwwww\nrbrwrwruuwwgbgubgwrgwuuwbuurgurggwbbwrguugrbrwrbrgugwrwgww\nbgwbrwbwruruwggubuuubububbbbrggubwuwbgugrbrburgwwbwwwww\nruubuwrwuubrbrrruwuuwruwwgggbrugrbrrwgwwgugrgrbuwbg\nrwwbbuubwwgguuubbwrgrbwwbrwwbbwwwbgbwbgwwbrrbww\nrbwrgwwwgwbbgwbwugrbrwwbgugbwubwbuurggbugguuugwg\nrrbbuugggwurwwugubburubbbbuggwwgburgwwubbrgww\ngggguwrguuwbwbrwwbbuwurgggggubrgbgbbrgrbrrrbbubgg\nggwubgwuwwgrbggbwgwrwbuguuwbubrrgwubwwbuwuuw\nrbugbrwuwwbguuwbwggrwrrrgwurbbbuwgugrubgrurbr\nrwbrugguuuruguubggggbuurburwwrwgwwbwrggbgugbwbgrbu\nrbrgwubguwuwbubruuwugubrgbwrugbwrgwrruwrrgw\nbuugurrbuuuwgwwggruuuuwwrbbuugwbgwbrbuuggwwgww\nugubururrwbugrbuuruwgwbwbuubguwwgbwrwgggggwgggub\nwugruubwwgrubwguwrgrwbubwbruwwbrgubugbrugurrggwgugbgww\nrbwgbuwgwrbugubwrgrbbuurwuurbgwgrwguwgwurwrgbrgwgrbwbrurw\nrruuwguuwurwuwggrbwwuurgrgbbruwwuwwrrwbugub\nbggbbubuggguwwugggwrgrgggbwwgwrwuburuguwbgrbu\nbguwgrrwgbggwguwggwwbwrggbugrubwwurrbrwwbuuwrurrrwrw\nburwwrguwrbrurgruwbwuwwuurwbbrruguguwbwbgrbwbuug\nwruugrgwbrgubbbbuuuwrgrgburgrgbwgbrugwrwrrrbrurwbg\nwrbuuwruguurgwbbrgwubbgwwuwrgbbrgwrbubggbwwgub\nrgrbwwurrwgwgwrrubwugwgwbgrggbrbrbbubwwgbbbuguubwu\nwwrgbgguwbgbururwwbrwwuwuwuuuurbbgwgggbwbbwubrrrggubwg\nrbuwgrbubrruguwuggrbuwuuwruuurruuwrrubgbwgg\nubbrwuubgrugrguguggrubrgurrrggubruuwbgwgrrburwggbwrrbgbwrgww\nwwrwrgggurbrwrwbbrbuguwbubgwgruguwgrrgubgggrgwubrgww\ngrwrwubgwuwwgwwwgbrburrgggbbwrwugwwrgubrbrubbggugurg\nugrgwggbrwrbbgrbrbuwgbgwrgbrgwwbruuguubwrbubrurwruubwwurwgww\nrrrrubgwwrwurgbuurrrbrrrbbruwwwwbgurwbugbbrrrbgww\nwgbuuugggburbwwggwbgugruggwbgbwugruwuwwwwgrwgbwuwr\nbububuubwgrrwrwrgubruwubbuubwrguggwugbgbgwgww\nrbgrbbugugwwwwubuugbwrruwbbubwbwwggugrbwgw\nrguggbwgbuubwbgbuwgbbrbwwurugbbuwwrwgrwuwgbbwguruwrb\nwbugurbbgwrrbuguggugwgwbwgwrburbwrugbrbrrwwbrrgwwgww\nbgbrwgbrrggwwwgwrbrbggwurrurbubwrrwgbrwgwugubburbgugbbr\nbbwrurbwbwugubwgrbbgbbwwbgrbgbwwbggwbruwbgrubbwrww\nuwurbrwwrruwgwrguwuwuubgwrgbbwgruwggrrgwrwwbbrbgbgbguwrbgr\nrggrbwrrrbgrbggguwuugbuubruwugbrrugwuuugwubb\nuugbwbbgwrbbggurgbbbbgwrrwbruurgwgwgbwuubgguuubrwgww\ngbwbbgrwwgugurgrggrbwwbwwrwgbbggwrbgwwgww\nwuurbgwgrwbrwwgwwbgbggggrubruuubgbbbruubrwgguurbgww\nubburbgurgguuwbruuurwwgburrrbwuwbgruwuburwbwbwrgbrbgww\nwbrbwgubuwubrrbugbuwrbbwrwbwwrrbwuruuwbuwbwrwburrrb\nugguuurburwubugrggburuwuuggwwbbwbrurwuuwbwbbgubw\nwrbugwggrbwgrrgbwggubgruwgggwggrrgrwwgrgwugbbuw\nrgbubwuugrwuwuwwrwurgrrubgrbbbbruuwgwuubrgr\nwwgrwuuwrbrwwbuuuurrruruuuurugrbrwwwrguwrwuggwuwwwburgwbb\ngwrrggbbggurwubggrurgwwwububggbguurbwwbgurwgrgww\nuwuurbbbuguubwuggrbwrububgwbgrrbrwbbgugrrwbrwrbrrrrwg\nguubggrguguwgbwrugurbrugruwrwbgbrwrgwwgurbruguubrbubr\nwgwbbrggbbggrbwbguubrgguwgwrbbgrruwbrrbbwgggugrgrgr\nwrgbrrrgwwbbrrgrgurrwbrgrggbrrgwbugrugbrwwbuwgww\nrbrggrrwgugubrrbrbbgwurbbrgwgubrrwwrwwurrurbwwgbu" ("PuzzleInput")) -> ("trimmed string"=w12:string)  [unwired: 1 in]
  n2 = call <userlib>:"Multi-line String to Array__ogtk.vi"("string"=w12) -> ("lines"=w11:string[])
  n3 = Split 1D Array(array=w11, index=2) -> (first subarray=w9:string[], second subarray=w4:string[])
  "Pattern" <- w4
  n4 = Concatenate Strings(w9) -> (w8:string)
  n5 = call <vilib>:"Trim Whitespace.vi"("string"=w8) -> ("trimmed string"=w3:string)  [unwired: 1 in]
  n6 = Spreadsheet String To Array(delimiter (Tab)=", ", format string="%s", spreadsheet string=w3, array type (2D Dbl)=string[] [] ("array")) -> (array=w5:string[])
  "array" <- w5
  n7 = Bundle By Name(cluster="object in", "Towels"=w5, "Pattern"=w4) -> (→"object out":refnum<class "2024_19.lvclass">)
  "Error Out" <- "Error In"
